vi "Compress.vi"(8 "error in (no error)":errorcluster, 11 "data":u8[](array[numeric])) -> (0 "error out":errorcluster, 2 "radio":dbl, 3 "compressed data":u8[](array[numeric]))   [LabVIEW 2020, in "GZip.lvclass"]
uses:
  GZip.lvclass
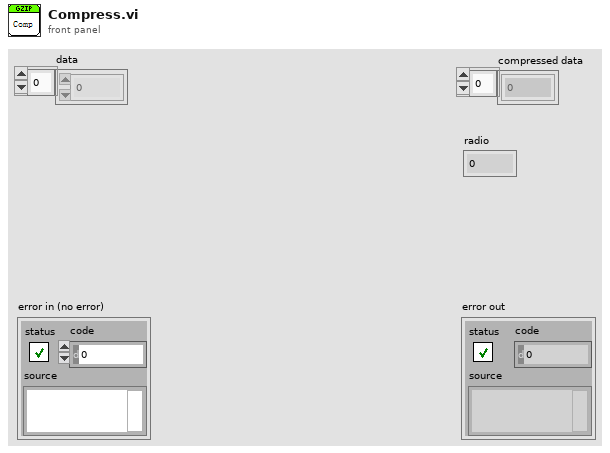
[diagram p1: front panel]
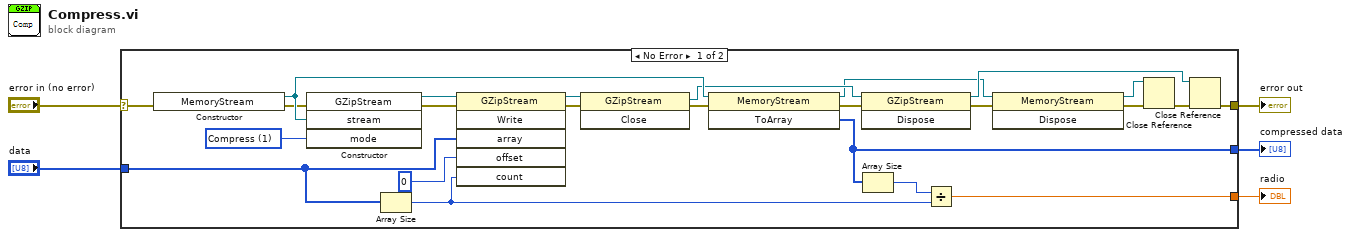
[diagram p0: block diagram]
diagram:
  n1 = case shown="No Error" "error in (no error)" {
    selector: "error in (no error)" -> [w18 w30]
    tunnel: [w13 w30] -> w4
    tunnel: [w9 _] -> w2
    tunnel: "data" -> [w8 _]
    tunnel: [w6 _] -> w1
    frame No Error {
      w20 = 1 items=["Decompress", "Compress"] ("mode")
      n2 = constructor class="MemoryStream"(error in=w18) -> (reference out=w23:refnum<k24>, error out=w19:errorcluster)  [unwired: 2 in, 1 out]
      n3 = constructor class="GZipStream"(error in=w19, "stream"=w23, "mode"=w20) -> (reference out=w21:refnum<k24>, error out=w22:errorcluster)  [unwired: 2 in, 3 out]
      n4 = Array Size(array=w8) -> (size(s)=w7:i32)
      n5 = invoke class="GZipStream" method="Write"(reference=w21, error in=w22, "array"=w8, "offset"=0, "count"=w7) -> (reference out=w28:refnum<k24>, error out=w24:errorcluster)  [unwired: 1 in, 4 out]
      n6 = invoke class="GZipStream" method="Close"(reference=w28, error in=w24) -> (reference out=w12:refnum<k24>, error out=w25:errorcluster)  [unwired: 1 in, 1 out]
      n7 = invoke class="MemoryStream" method="ToArray"(reference=w23, error in=w25) -> (reference out=w11:refnum<k24>, error out=w29:errorcluster, "ToArray"=w6:u8[])  [unwired: 1 in]
      n8 = invoke class="GZipStream" method="Dispose"(reference=w12, error in=w29) -> (reference out=w14:refnum<k24>, error out=w27:errorcluster)  [unwired: 1 in, 1 out]
      n9 = Array Size(array=w6) -> (size(s)=w10:i32)
      n10 = Divide(x=w10, y=w7) -> (x/y=w9:dbl)
      n11 = invoke class="MemoryStream" method="Dispose"(reference=w11, error in=w27) -> (reference out=w16:refnum<k24>, error out=w17:errorcluster)  [unwired: 1 in, 1 out]
      n12 = Close Reference(reference=w16, error in (no error)=w17) -> (error out=w15:errorcluster)
      n13 = Close Reference(reference=w14, error in (no error)=w15) -> (error out=w13:errorcluster)
    }
    frame Error {
    }
  }
  "error out" <- w4
  "radio" <- w2
  "compressed data" <- w1
